vi "NI_PCIE_6509.vi"(11 "Queue Ref In":T1={"UI"=refnum, "Message"=refnum, "Data"=refnum, "Caller"=refnum, "Name"="000 Common", "Data Path"=path "", "Class Path"=path "", "SubPanel"=refnum, "Project Name"="", "MNT"="", "Title"="", "Data Source"=refnum, "Queue List"={}, "VI"=refnum, "UE"=refnum}) -> ()   [LabVIEW 2020]
doc: "PCIE_6509"
uses:
  Alin/QMH/000 Module Data Type.ctl
  Alin/QMH/Queue Message.ctl
  9999 SubVI/Global/Data Global/SDQ Data Type.ctl
  <vilib>/DAQmx/read.llb/DAQmx Read (Digital 1D Bool NChan 1Samp 1Line).vi
  <vilib>/DAQmx/create/channels.llb/DAQmx Create Channel (DI-Digital Input).vi
  <vilib>/DAQmx/miscellaneous.llb/DAQmx Fill In Error Info.vi
  <resource>/objmgr/daqmx.rc
panel:
  out "Type":map{string, string}(c390)
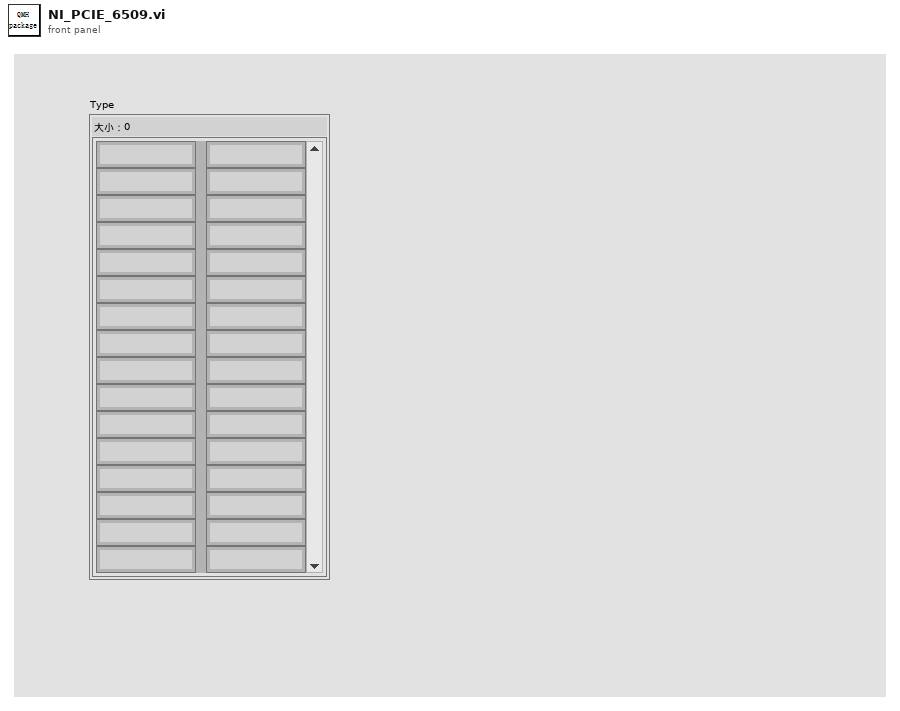
[diagram p1: front panel]
types:
  T1 = typedef "000 Module Data Type.ctl" = cluster{"UI":refnum<queue>, "Message":refnum<queue>, "Data":refnum<queue>, "Caller":refnum<queue>, "Name":string, "Data Path":path, "Class Path":path, "SubPanel":refnum<vi>, "Project Name":string, "MNT":string, "Title":string, "Data Source":refnum<queue>, "Queue List":map{string, refnum<queue>}, "VI":refnum<vi>, "UE":refnum<user-event>}
  T2 = typedef "SDQ Data Type.ctl" = cluster{"CAN Length":string, "CAN Name":string, "CAN ID":string, "CAN Type":string, "Test Item":string, "Byte Order":string, "Instruction":string, "Control Type":string, "Group":string, "Offset":dbl, "Coefficient":dbl, "Write Enable":bool, "Lable Type":string, "Key?":string, "Set Value":string, "Upper":dbl, "Lower":dbl, "Unit":string, "Formula":string, "Test Item Type":string, "Length":i32, "Address":string, "Name":string, "Identifier":string, "Data Type":string, "Enumerate?":string, "Enumerate List":string, "Data":string, "Source":string}
  T3 = cluster{"Queue":T1, "Delay":cluster{"Count Time(ms)":u32, "Delay Time(ms)":u32, "Next":string}, "Data":map{string, T2}, "PCIE_6509":cluster{"Port":string, "Task":refnum<k21>}, "IDS":string[], "Type":map{string, string}}
  T4 = typedef "005 Data Source Type.ctl" = cluster{"Device Name":string, "Device Model":string, "Device Driver":string, "IP Address":string, "Port":string, "Remark":string, "Enable":string, "Path":string}
  T5 = cluster{"Name":string, "Type":map{string, string}}
  T6 = typedef "eventvkey.ctl" = enum16{"ASCII", "Enter", "Return", "Shift", "Ctrl", "Alt", "Cmd", "Opt", "Caps", "NumLock", "Clear", "Break", "Up", "Down", "Left", "Right", "Insert", "Delete", "Home", "End", "PageUp", "PageDown", "Escape", "Help", "Pause", "ScrollLock", "F1", "F2", "F3", "F4", "F5", "F6", "F7", "F8", "F9", "F10", "F11", "F12", "F13", "F14", "F15", "F16", "F17", "F18", "F19", "F20", "F21", "F22", "F23", "F24", "Play", "VolumeUp", "VolumeDown", "Mute", "Two Byte Char"}
  T7 = cluster{"Shift":bool, "Ctrl":bool, "Alt":bool, "Cmd":bool, "Opt":bool}
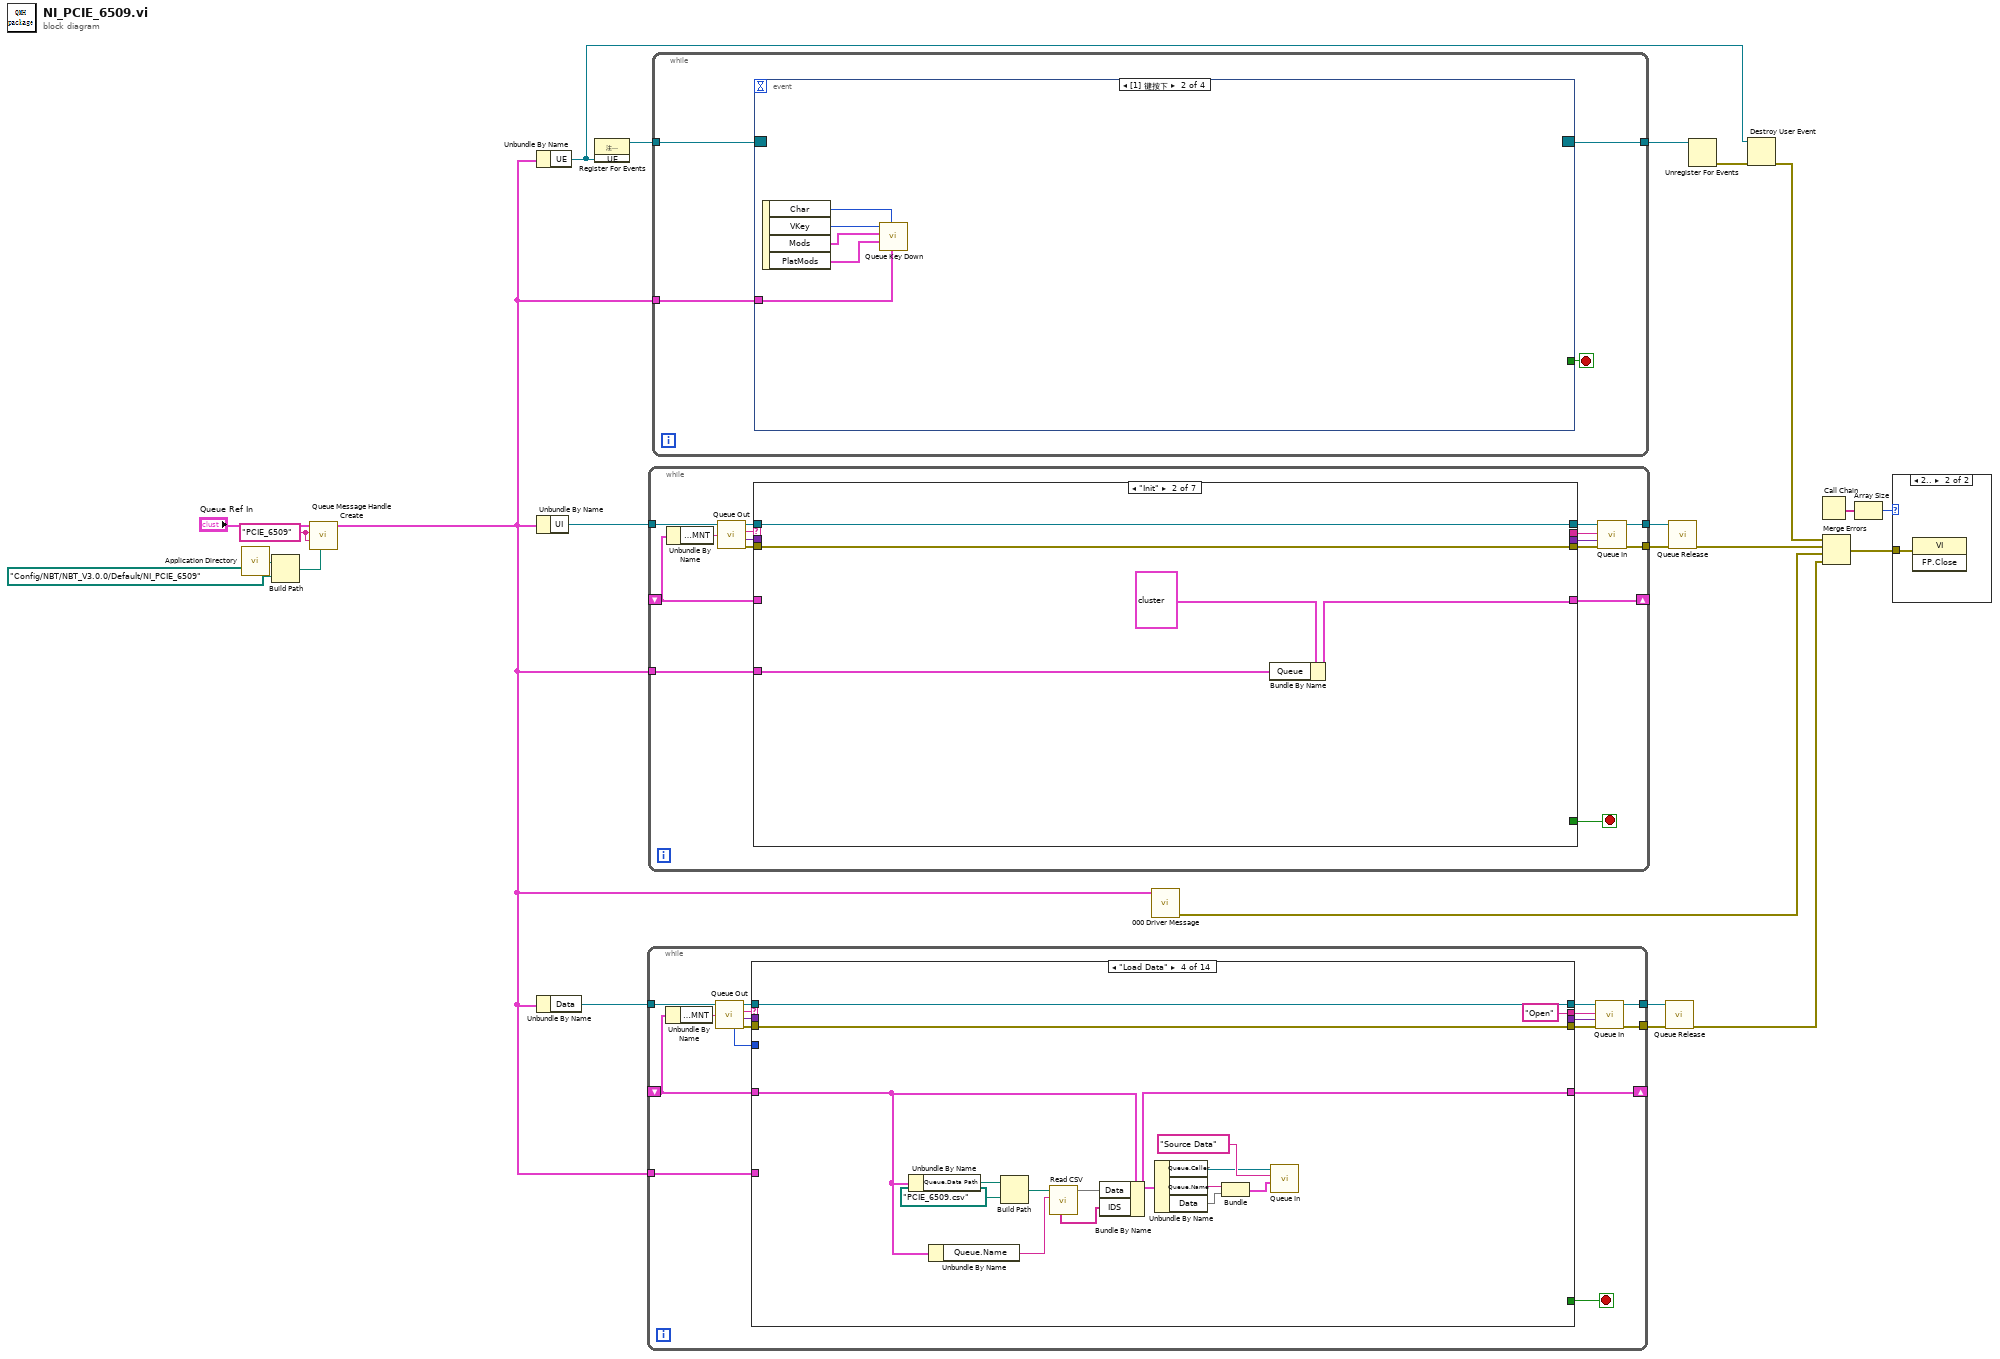
[diagram p0: block diagram]
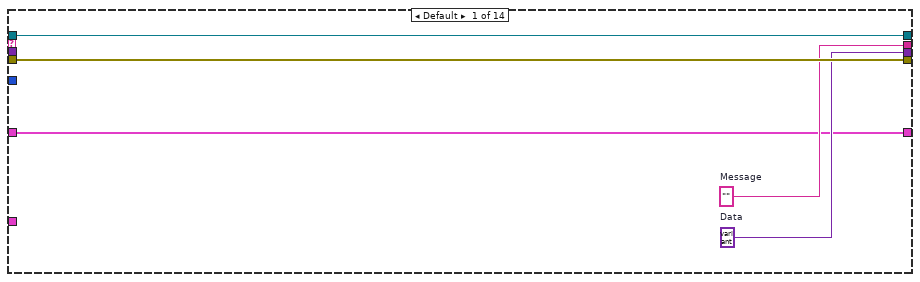
[diagram p2: hidden frame]
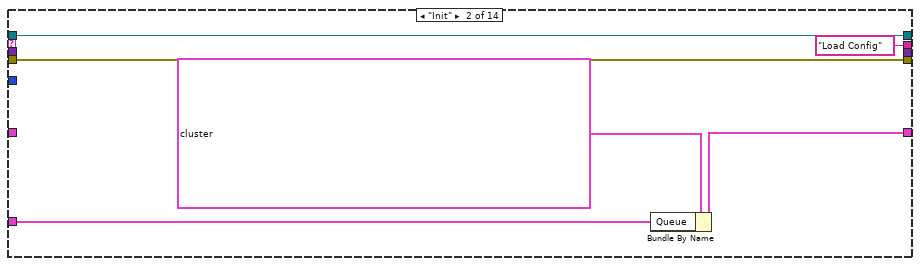
[diagram p3: hidden frame]
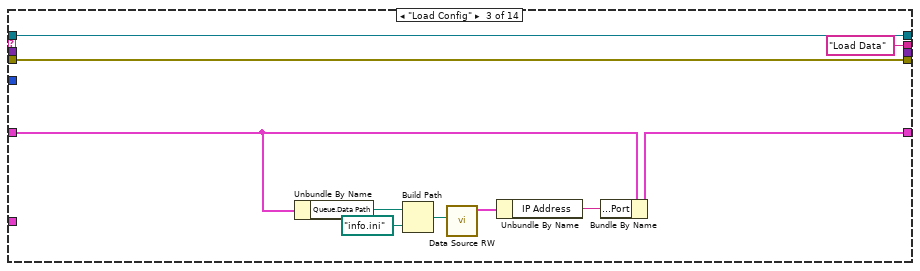
[diagram p4: hidden frame]
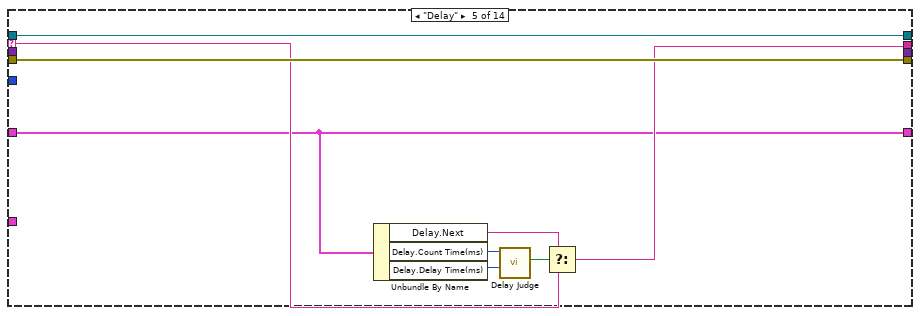
[diagram p5: hidden frame]
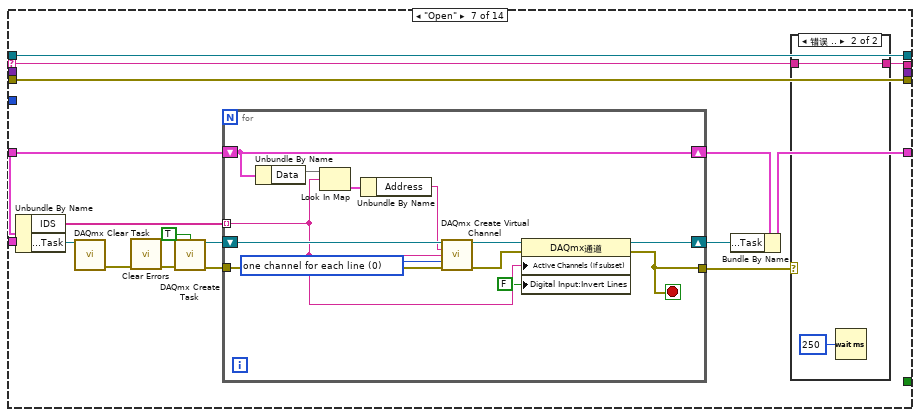
[diagram p7: hidden frame]
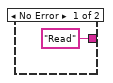
[diagram p8: hidden frame]
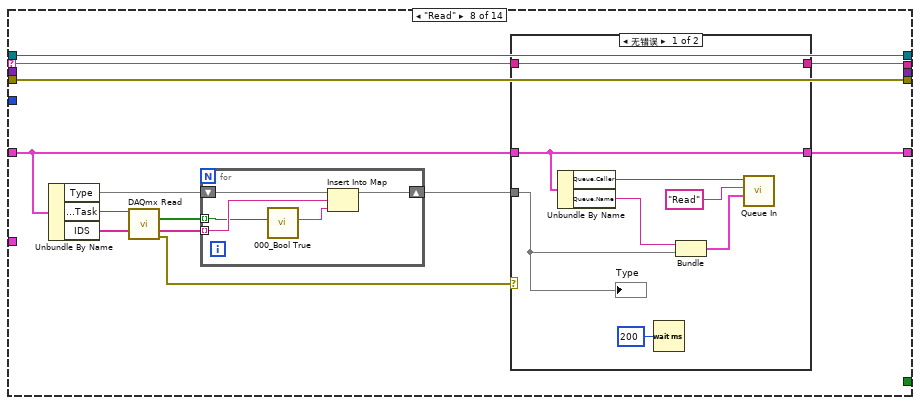
[diagram p9: hidden frame]
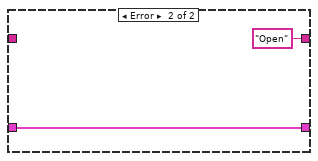
[diagram p10: hidden frame]
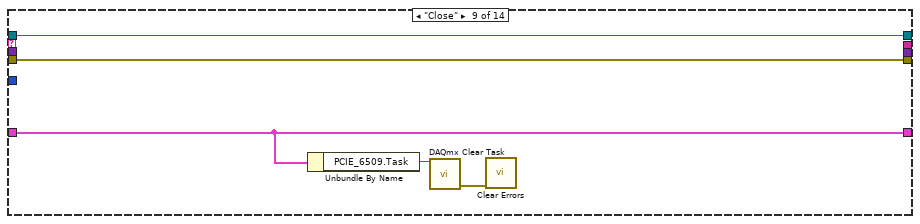
[diagram p11: hidden frame]
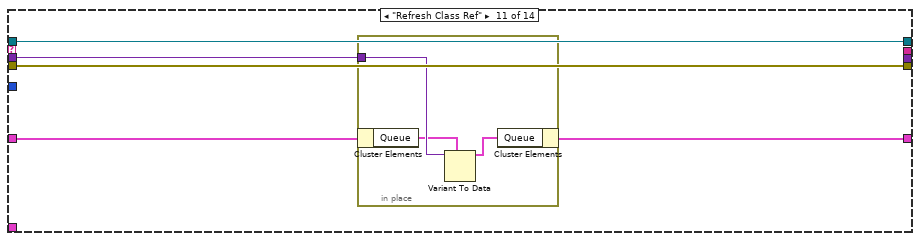
[diagram p13: hidden frame]
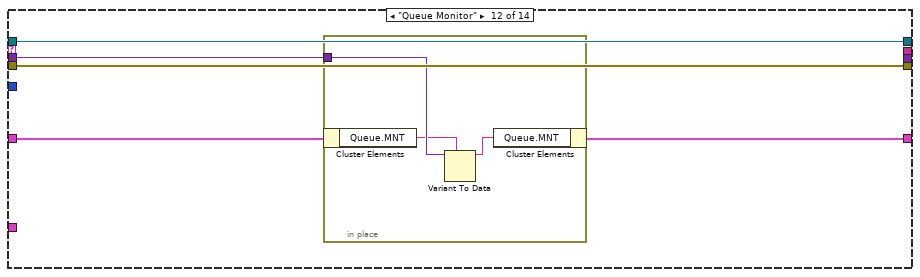
[diagram p14: hidden frame]
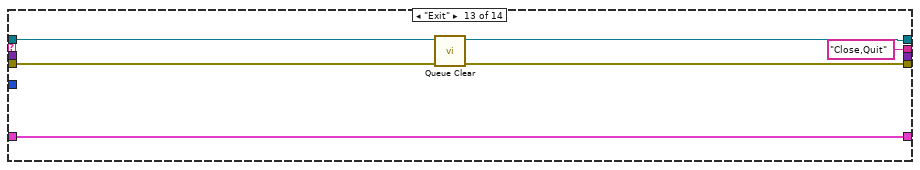
[diagram p15: hidden frame]
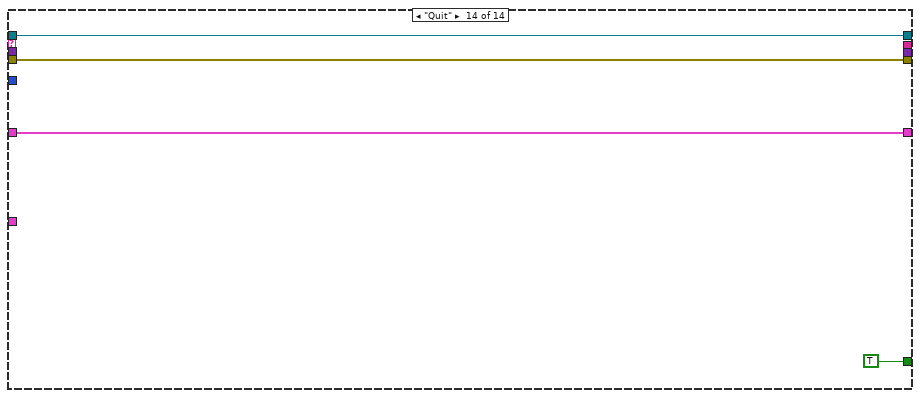
[diagram p16: hidden frame]
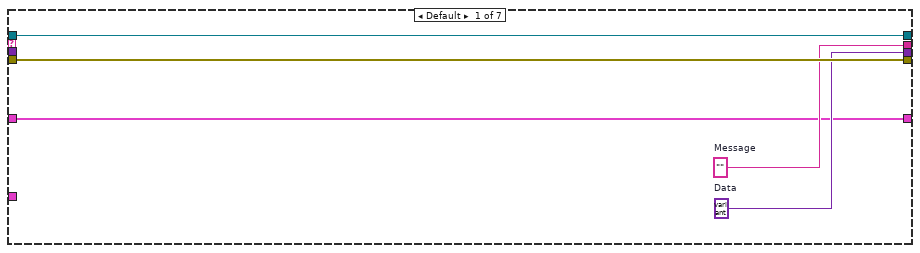
[diagram p18: hidden frame]
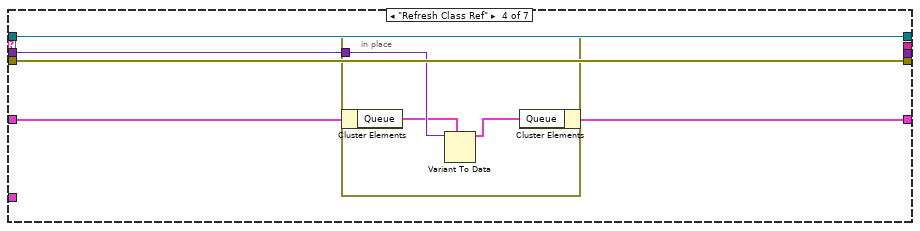
[diagram p20: hidden frame]
diagram:
  w1 = "PCIE_6509" ("Title")
  n1 = call <vilib>:"Application Directory.vi"() -> ("Application Directory"=w4:path)
  n2 = Build Path(base path=w4, name or relative path=path "Config/NBT/NBT_V3.0.0/Default/NI_PCIE_6509" ("名称或相对路径")) -> (appended path=w2:path)
  n3 = call "Queue Message Handle Create.vi"("Data Path"=w2, "Name"=w1, "Title"=w1, "Queue Ref In"="Queue Ref In") -> ("Queue Ref Out"=w5:T1)  [unwired: 6 in, 1 out]
  n4 = Unbundle By Name(w5) -> ("UE"=w7:refnum<user-event>)
  n5 = Unbundle By Name(w5) -> ("UI"=w18:refnum<queue>)
  n6 = Unbundle By Name(w5) -> ("Data"=w10:refnum<queue>)
  n7 = register-events(w7) -> (reference out=w23:refnum<event-registration>)  [unwired: 2 in, 1 out]
  n8 = while {
    tunnel: w10 -> [w36]
    tunnel: [w33] -> w12
    tunnel: [w32] -> w11
    shift-right: [w28] -> _
    shift-left: _ -> [w25]
    tunnel: w5 -> [w24]
    stop <- w40 stop-if-true
    n9 = Unbundle By Name(w25) -> ("Queue.MNT"=w26:string)
    n10 = call "Queue Out.vi"("Monitor"=w26, "Queue In"=w36) -> ("error out"=w39:errorcluster, "Data"=w37:variant, "Message"=w38:string, "Queue Out"=w35:refnum<queue>, "Queue NUmber"=w27:i32)  [unwired: 5 in]
    n11 = case shown="\"Load Data\"" w38 {
      selector: w38 -> [_ _ _ _ w79 _ w95 w126 _ _ _ _ _ _]
      tunnel: w35 -> [w45 w51 w61 w77 w86 w89 w105 w133 w153 w156 w161 w169 w177 w181]
      tunnel: w39 -> [w44 w50 w60 w76 w85 w88 w104 w132 w152 w155 w160 w168 w175 w182]
      tunnel: [w45 w51 w61 w77 w86 w89 w105 w133 w153 w156 w161 w169 w176 w181] -> w34
      tunnel: [w44 w50 w60 w76 w85 w88 w104 w132 w152 w155 w160 w168 w174 w182] -> w31
      tunnel: [w43 "Load Config" ("Next") "Load Data" ("Next") "Open" ("Next") w80 _ w94 w125 _ _ _ _ "Close,Quit" _] -> w30
      tunnel: [_ _ _ _ _ _ _ _ _ _ _ _ _ TRUE] -> w40
      tunnel: [w42 _ _ _ _ _ _ _ _ _ _ _ _ _] -> w29
      tunnel: w37 -> [_ _ _ _ _ _ _ _ _ _ w157 w165 _ _]
      tunnel: [w41 w47 w53 w66 w78 w87 w102 w127 w151 w154 w158 w166 w173 w179] -> w28
      tunnel: w25 -> [w41 _ w58 w63 w78 w87 w92 w128 w151 w154 w159 w167 w173 w179]
      tunnel: w27 -> [_ _ _ _ _ _ _ _ _ _ _ _ _ _]
      tunnel: w24 -> [_ w46 _ _ _ _ _ _ _ _ _ _ _ _]
      frame Default {
        w42 = variant  # Data
        w43 = ""  # Message
      }
      frame "Init" {
        n12 = Bundle By Name(cluster=T3 {"Queue"={"UI"=refnum, "Message"=refnum, "Data"=refnum, "Caller"=refnum, "Name"="000 Common", "Data Path"=path "", "Class Path"=path "", "SubPanel"=refnum, "Project Name"="", "MNT"="", "Title"="", "Data Source"=refnum, "Queue List"={}, "VI"=refnum, "UE"=refnum}, "Delay"={"Count Time(ms)"=250, "Delay Time(ms)"=250, "Next"="Receive Data,Delay"}, "Data"={}, "PCIE_6509"={"Port"="", "Task"=""}, "IDS"=[], "Type"={}}, "Queue"=w46) -> (w47:T3)
      }
      frame "Load Config" {
        n13 = Unbundle By Name(w58) -> ("Queue.Data Path"=w57:path)
        n14 = Build Path(base path=w57, name or relative path=path "info.ini" ("名称或相对路径")) -> (appended path=w55:path)
        n15 = call "Data Source RW.vi"("Source Path"=w55) -> ("Data Type Out"=w54:T4)  [unwired: 7 in, 3 out]
        n16 = Unbundle By Name(w54) -> ("IP Address"=w52:string)
        n17 = Bundle By Name(cluster=w58, "PCIE_6509.Port"=w52) -> (w53:T3)
      }
      frame "Load Data" {
        n18 = Unbundle By Name(w63) -> ("Queue.Data Path"=w75:path)
        n19 = Unbundle By Name(w63) -> ("Queue.Name"=w62:string)
        n20 = Build Path(base path=w75, name or relative path=path "PCIE_6509.csv" ("名称或相对路径")) -> (appended path=w73:path)
        n21 = call "Read CSV.vi"("Source"=w62, "Data Path"=w73) -> (3:"Identifiers Out"=w72:map{string, T2}, 6:"Identifiers Out"=w65:string[])  [unwired: 2 in, 6 out]
        n22 = Bundle By Name(cluster=w63, "Data"=w72, "IDS"=w65) -> (w66:T3)
        n23 = Unbundle By Name(w66) -> ("Queue.Caller"=w67:refnum<queue>, "Queue.Name"=w71:string, "Data"=w69:map{string, T2})
        n24 = Bundle("Name"=w71, "Data"=w69) -> (w70:cluster{"Name":string, "Data":map{string, T2}})  [unwired: 1 in]
        n25 = call "Queue In.vi"("Data"=w70, "Message"="Source Data", "Queue In"=w67) -> ()  [unwired: 7 in, 2 out]
      }
      frame "Delay" {
        n26 = Unbundle By Name(w78) -> ("Delay.Next"=w84:string, "Delay.Count Time(ms)"=w81:u32, "Delay.Delay Time(ms)"=w82:u32)
        n27 = call "Delay Judge.vi"("Delay Time(ms)"=w82, "Count Time(ms)"=w81) -> ("Time Out?"=w83:bool)  [unwired: 5 in, 4 out]
        n28 = Select(t=w84, s=w83, f=w79) -> (s? t:f=w80:string)
      }
      frame "===Driver====" {
      }
      frame "Open" {
        n29 = Unbundle By Name(w92) -> ("IDS"=w93:string[], "PCIE_6509.Task"=w101:refnum<k21>)
        n30 = call <vilib>:"DAQmx Clear Task.vi"("task in"=w101) -> ("error out"=w100:errorcluster)  [unwired: 14 in]
        n31 = call <vilib>:"Clear Errors.vi"("error in (no error)"=w100) -> ("error out"=w99:errorcluster)  [unwired: 5 in, 1 out]
        n32 = call <vilib>:"DAQmx Create Task.vi"("auto cleanup"=TRUE, "error in"=w99) -> ("task out"=w98:refnum<k21>, "error out"=w90:errorcluster)  [unwired: 12 in]
        n33 = for {
          shift-right: [w114] -> w97
          shift-left: w98 -> [w121]
          tunnel: [w112] -> w96
          tunnel: w93 -> [w111] mode=indexing
          shift-right: [w120] -> w91
          shift-left: w92 -> [w120]
          tunnel: w90 -> [w116]
          stop <- w112 stop-if-true
          w110 = 0 items=["one channel for each line", "one channel for all lines"] ("line grouping")
          n34 = Unbundle By Name(w120) -> ("Data"=w119:map{string, T2})
          n35 = Look In Map(map=w119, key=w111) -> (value=w118:T2)  [unwired: 1 in, 1 out]
          n36 = Unbundle By Name(w118) -> ("Address"=w117:string)
          n37 = call-poly <vilib>:"DAQmx Create Virtual Channel.vi"("task in"=w121, "lines"=w117, "name to assign"=w111, "line grouping"=w110, "error in"=w116) -> ("task out"=w115:refnum<k21>, "error out"=w113:errorcluster)  [unwired: 9 in]
          n38 = property class="DAQmx通道"(reference=w115, error in=w113, "Active Channels (if subset)"=w111, "Digital Input:Invert Lines"=FALSE ("DI.InvertLines")) -> (reference out=w114:refnum<k21>, error out=w112:errorcluster)
        }
        n39 = Bundle By Name(cluster=w91, "PCIE_6509.Task"=w97) -> (w102:T3)
        n40 = case shown="错误 .." w96 {
          tunnel: w95 -> [_ w108]
          tunnel: ["Read" w108] -> w94
          frame No Error {
          }
          frame Error {
            n41 = Wait (ms)(milliseconds to wait=u32 250 ("等待时间（毫秒）")) -> ()  [unwired: 1 out]
          }
        }
      }
      frame "Read" {
        n42 = Unbundle By Name(w128) -> ("Type"=w130:map{string, string}, "PCIE_6509.Task"=w124:refnum<k21>, "IDS"=w131:string[])
        n43 = call-poly <vilib>:"DAQmx Read.vi"("task/channels in"=w124) -> ("data"=w123:bool[], "error out"=w122:errorcluster)  [unwired: 12 in, 1 out]
        n44 = for {
          tunnel: w131 -> [w147] mode=indexing
          shift-right: [w145] -> w129
          shift-left: w130 -> [w148]
          tunnel: w123 -> [w144] mode=indexing
          n45 = call "000_Bool True.vi"("Value"=w144) -> ("String Out"=w146:string)  [unwired: 9 in, 1 out]
          n46 = Insert Into Map(map in=w148, key=w147, value=w146) -> (map out=w145:map{string, string})  [unwired: 2 out]
        }
        n47 = case shown="无错误" w122 {
          tunnel: w129 -> [w134 _]
          tunnel: w128 -> [w141 w143]
          tunnel: [w141 w143] -> w127
          tunnel: w126 -> [w136 _]
          tunnel: [w136 "Open"] -> w125
          frame No Error {
            n48 = Unbundle By Name(w141) -> ("Queue.Caller"=w140:refnum<queue>, "Queue.Name"=w138:string)
            n49 = Wait (ms)(milliseconds to wait=u32 200 ("等待时间（毫秒）")) -> ()  [unwired: 1 out]
            n50 = Bundle("Name"=w138, "Type"=w134) -> (w137:T5)  [unwired: 1 in]
            n51 = call "Queue In.vi"("Data"=w137, "Message"="Read", "Queue In"=w140) -> ()  [unwired: 7 in, 2 out]
            "Type" <- w134
          }
          frame Error {
          }
        }
      }
      frame "Close" {
        n52 = Unbundle By Name(w151) -> ("PCIE_6509.Task"=w150:refnum<k21>)
        n53 = call <vilib>:"DAQmx Clear Task.vi"("task in"=w150) -> ("error out"=w149:errorcluster)  [unwired: 14 in]
        n54 = call <vilib>:"Clear Errors.vi"("error in (no error)"=w149) -> ()  [unwired: 5 in, 2 out]
      }
      frame "====System====" {
      }
      frame "Refresh Class Ref" {
        n55 = in-place {
          in-place-border: w157 -> [w164]
          n56 = in-place-cluster #1(w159) -> ("Queue"=w163:T1)
          n57 = Variant To Data(type=w163, Variant=w164) -> (data=w162:T1)  [unwired: 1 in, 1 out]
          n58 = in-place-cluster #1("Queue"=w162) -> (w158:T3)
        }
      }
      frame "Queue Monitor" {
        n59 = in-place {
          in-place-border: w165 -> [w172]
          n60 = in-place-cluster #2(w167) -> ("Queue.MNT"=w171:string)
          n61 = Variant To Data(type=w171, Variant=w172) -> (data=w170:string)  [unwired: 1 in, 1 out]
          n62 = in-place-cluster #2("Queue.MNT"=w170) -> (w166:T3)
        }
      }
      frame "Exit" {
        n63 = call "Queue Clear.vi"("error in (no error)"=w175, "Queue In"=w177) -> ("error out"=w174:errorcluster, "Queue Out"=w176:refnum<queue>)  [unwired: 8 in]
      }
      frame "Quit" {
      }
    }
    n64 = call "Queue In.vi"("error in (no error)"=w31, "Data"=w29, "Message"=w30, "Queue In"=w34) -> ("error out"=w32:errorcluster, "Queue Out"=w33:refnum<queue>)  [unwired: 6 in]
  }
  n65 = while {
    tunnel: w18 -> [w194]
    tunnel: [w191] -> w20
    tunnel: [w190] -> w19
    shift-right: [w186] -> _
    shift-left: _ -> [w185]
    tunnel: w5 -> [w183]
    stop <- w198 stop-if-true
    n66 = Unbundle By Name(w185) -> ("Queue.MNT"=w184:string)
    n67 = call "Queue Out.vi"("Monitor"=w184, "Queue In"=w194) -> ("error out"=w197:errorcluster, "Data"=w195:variant, "Message"=w196:string, "Queue Out"=w193:refnum<queue>)  [unwired: 5 in, 1 out]
    n68 = case shown="\"Init\"" w196 {
      selector: w196 -> [_ _ _ _ _ w230 _]
      tunnel: w193 -> [w203 w208 w211 w216 w224 w237 w243]
      tunnel: w197 -> [w202 w207 w210 w215 w223 w235 w244]
      tunnel: [w203 w208 w211 w216 w224 w236 w243] -> w192
      tunnel: [w202 w207 w210 w215 w223 w234 w244] -> w189
      tunnel: [w201 _ _ _ _ "Quit" _] -> w188
      tunnel: [_ _ _ _ _ _ TRUE] -> w198
      tunnel: [w200 _ _ _ _ _ _] -> w187
      tunnel: w195 -> [_ _ _ w212 w220 _ _]
      tunnel: [w199 w205 w209 w213 w221 w229 w241] -> w186
      tunnel: w185 -> [w199 _ w209 w214 w222 w229 w241]
      tunnel: w183 -> [_ w204 _ _ _ _ _]
      frame Default {
        w200 = variant  # Data
        w201 = ""  # Message
      }
      frame "Init" {
        n69 = Bundle By Name(cluster=cluster{"Queue":T1} {"Queue"={"UI"=refnum, "Message"=refnum, "Data"=refnum, "Caller"=refnum, "Name"="000 Common", "Data Path"=path "", "Class Path"=path "", "SubPanel"=refnum, "Project Name"="", "MNT"="", "Title"="", "Data Source"=refnum, "Queue List"={}, "VI"=refnum, "UE"=refnum}}, "Queue"=w204) -> (w205:cluster{"Queue":T1})
      }
      frame "====System====" {
      }
      frame "Refresh Class Ref" {
        n70 = in-place {
          in-place-border: w212 -> [w219]
          n71 = in-place-cluster #3(w214) -> ("Queue"=w218:T1)
          n72 = Variant To Data(type=w218, Variant=w219) -> (data=w217:T1)  [unwired: 1 in, 1 out]
          n73 = in-place-cluster #3("Queue"=w217) -> (w213:cluster{"Queue":T1})
        }
      }
      frame "Queue Monitor" {
        n74 = in-place {
          in-place-border: w220 -> [w227]
          n75 = in-place-cluster #4(w222) -> ("Queue.MNT"=w226:string)
          n76 = Variant To Data(type=w226, Variant=w227) -> (data=w225:string)  [unwired: 1 in, 1 out]
          n77 = in-place-cluster #4("Queue.MNT"=w225) -> (w221:cluster{"Queue":T1})
        }
      }
      frame "Exit" {
        n78 = Unbundle By Name(w229) -> ("Queue.Message"=w233:refnum<queue>, "Queue.Data"=w232:refnum<queue>, "Queue.UE"=w228:refnum<user-event>)
        n79 = Build Array(w233, w232) -> (w231:refnum<queue>[])
        n80 = Generate User Event(user event=w228, event data cluster=w230) -> ()  [unwired: 2 in, 2 out]
        n81 = for {
          tunnel: w231 -> [w240] mode=indexing
          tunnel: w230 -> [w239]
          n82 = call "Queue In.vi"("Message"=w239, "Queue In"=w240) -> ()  [unwired: 8 in, 2 out]
        }
        n83 = call "Queue Clear.vi"("error in (no error)"=w235, "Queue In"=w237) -> ("error out"=w234:errorcluster, "Queue Out"=w236:refnum<queue>)  [unwired: 8 in]
      }
      frame "Quit" {
      }
    }
    n84 = call "Queue In.vi"("error in (no error)"=w189, "Data"=w187, "Message"=w188, "Queue In"=w192) -> ("error out"=w190:errorcluster, "Queue Out"=w191:refnum<queue>)  [unwired: 6 in]
  }
  n85 = while {
    tunnel: w23 -> [w248]
    tunnel: [w246] -> w22
    tunnel: w5 -> [w245]
    stop <- w247 stop-if-true
    n86 = event shown="[1] 键按下" {
      selector: w248 -> [_ _ _ _]
      dyn-events: [_ _ _ _] -> w246
      timeout: _ -> [_ _ _ _]
      tunnel: [_ _ w254 _] -> w247
      tunnel: w245 -> [_ w249 _ w259]
      event Timeout {
        n87 = event-data() -> ()  [unwired: 1 in, 1 out]
      }
      event Key Down {
        n88 = event-data() -> ("Char"=w253:i16, "VKey"=w252:T6, "Mods"=w251:cluster{"Num Pad":bool, "Menu Key":bool}, "PlatMods"=w250:T7)  [unwired: 1 in]
        n89 = call "Queue Key Down.vi"("Queue Ref Out"=w249, "C"=w253, "Platform Key"=w250, "Group Key"=w251, "V Key"=w252) -> ()  [unwired: 6 in, 1 out]
      }
      event User Event {
        n90 = event-data() -> ("Message"=w256:string)  [unwired: 1 in]
        n91 = Equal?(x=w256, y="Exit") -> (x = y?=w254:bool)
      }
      event Panel Close? {
        n92 = event-data() -> ()  [unwired: 1 in, 1 out]
        n93 = Call Chain() -> (call chain=w261:string[])
        n94 = Array Size(array=w261) -> (size(s)=w260:i32)
        n95 = case shown="2, 默认" w260 {
          tunnel: w259 -> [w265 w268]
          tunnel: [w264 w267] -> w258
          tunnel: ["Panel Hidden" ("Message") "Exit Prepare" ("Message")] -> w257
          frame 2, Default {
            n96 = Unbundle By Name(w265) -> ("Message"=w264:refnum<queue>)
          }
          frame 1 {
            n97 = Unbundle By Name(w268) -> ("Message"=w267:refnum<queue>)
          }
        }
        n98 = call "Queue In.vi"("Message"=w257, "Queue In"=w258) -> ()  [unwired: 8 in, 2 out]
        n99 = event-data("Discard?"=TRUE ("放弃？")) -> ()  [unwired: 1 in, 1 out]
      }
    }
  }
  n100 = call "000 Driver Message.vi"("Queue In"=w5) -> ("error out"=w8:errorcluster)  [unwired: 8 in, 2 out]
  n101 = call "Queue Release.vi"("error in (no error)"=w11, "Queue In"=w12) -> ("error out"=w9:errorcluster)  [unwired: 9 in]
  n102 = call "Queue Release.vi"("error in (no error)"=w19, "Queue In"=w20) -> ("error out"=w16:errorcluster)  [unwired: 9 in]
  n103 = Unregister For Events(event registration refnum=w22) -> (error out=w21:errorcluster)  [unwired: 1 in]
  n104 = Destroy User Event(user event=w7, error in=w21) -> (error out=w17:errorcluster)
  n105 = Call Chain() -> (call chain=w14:string[])
  n106 = Merge Errors(w17, w16, w8, w9) -> (w15:errorcluster)
  n107 = Array Size(array=w14) -> (size(s)=w13:i32)
  n108 = case shown="2.." w13 {
    tunnel: w15 -> [_ w269]
    frame 0, Default {
    }
    frame 2.. {
      n109 = invoke class="VI" method="FP.Close"(error in=w269) -> ()  [unwired: 2 in, 3 out]
    }
  }
